vi "xijk_image_read.vi"(8 "error in (no error)":errorcluster, 11 "path in":path=path "H:/Programming/+ Labview/08 spectrum analyzer/example images/7666d8daad.jpg") -> (0 "error out":errorcluster, 3 "path out":path)   [LabVIEW 2010, in "xijk_combined_file.lvlib"]
uses:
  xijk_combined_file.lvlib
  <vilib>/Utility/file.llb/Write To Spreadsheet File (DBL).vi
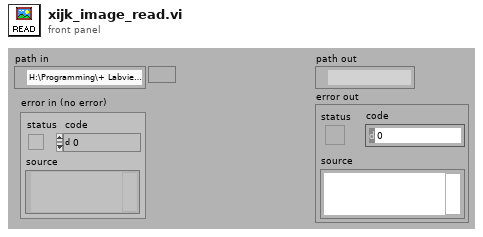
[diagram p1: front panel]
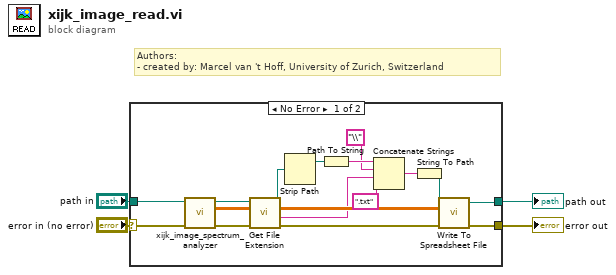
[diagram p0: block diagram]
diagram:
  # "Authors: \n- created by: Marcel van 't Hoff, University of Zurich, Switzerland"
  n1 = case shown="No Error" "error in (no error)" {
    selector: "error in (no error)" -> [w19 w21]
    tunnel: "path in" -> [w7 w20]
    tunnel: [w17 w20] -> w3
    tunnel: [w18 w21] -> w2
    frame No Error {
      n2 = call "xijk_image_spectrum_analyzer.vi"("error in (no error)"=w19, "Start Path"=w7) -> ("error out"=w5:errorcluster, "array out"=w16:dbl[][], "path out"=w6:path)  [unwired: 7 in]
      n3 = call <vilib>:"Get File Extension.vi"("error in (no error)"=w5, "file"=w6) -> ("error out"=w18:errorcluster, "filename without extension"=w15:string, "dup file"=w11:path)  [unwired: 6 in, 1 out]
      n4 = Strip Path(path=w11) -> (stripped path=w10:path)  [unwired: 1 out]
      n5 = Path To String(path=w10) -> (string=w9:string)
      n6 = Concatenate Strings(w9, "\\" ("string"), w15, ".txt" ("name or relative path")) -> (w13:string)
      n7 = String To Path(string=w13) -> (path=w12:path)
      n8 = call-poly <vilib>:"Write To Spreadsheet File.vi"("2D data"=w16, "file path (dialog if empty)"=w12) -> ("new file path (Not A Path if cancelled)"=w17:path)  [unwired: 6 in]
    }
    frame Error {
    }
  }
  "path out" <- w3
  "error out" <- w2
